vi "Get Table Data.vi"(7 "Count? (F)":bool, 8 "error in (no error)":errorcluster, 9 "Column Conditions[] (Optional)":T1[](array[typedef]), 10 "Header Order[] (Optional)":string[](array[string]), 11 "SLL Table in":refnum<class "SLL Table.lvclass">) -> (0 "error out":errorcluster, 1 "2D Data Out[][]":string[][](array[string]), 2 "Headers Out[]":string[](array[string]), 3 "SLL Table out":refnum<class "SLL Table.lvclass">)   [LabVIEW 2014, in "SLL Table.lvclass"]
doc: "Get the data that you need & in the column order you want. \n\nYou can specify the column header and the value as conditions."
uses:
  SLL Table.lvclass
  _Typedefs/ColumnConditionCluster.ctl
  <userlib>/_OpenG.lib/array/array.llb/Remove Duplicates from 1D Array (String)__ogtk.vi
  SLL String/SLL String.lvlib
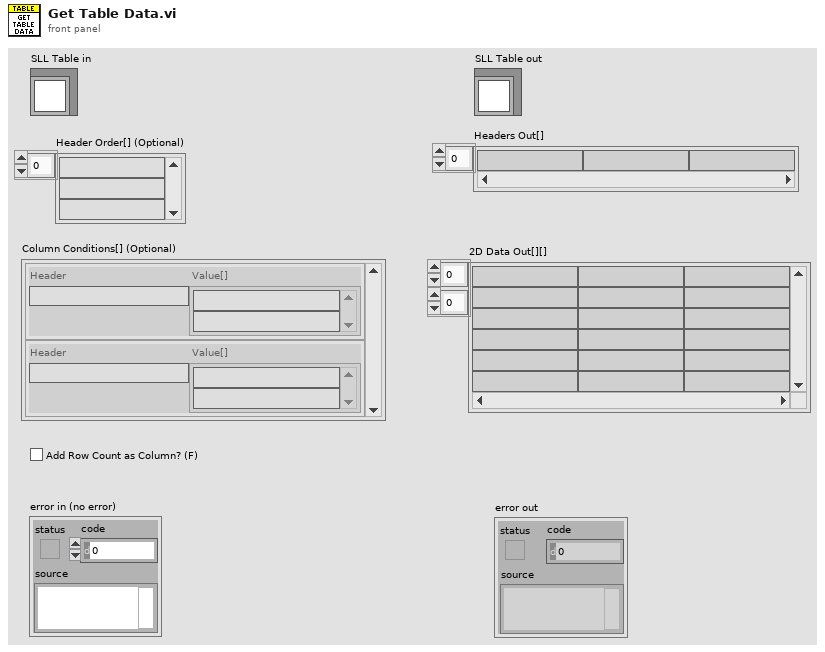
[diagram p1: front panel]
types:
  T1 = typedef "ColumnConditionCluster.ctl" = cluster{"Header":string, "Value[]":string[]}
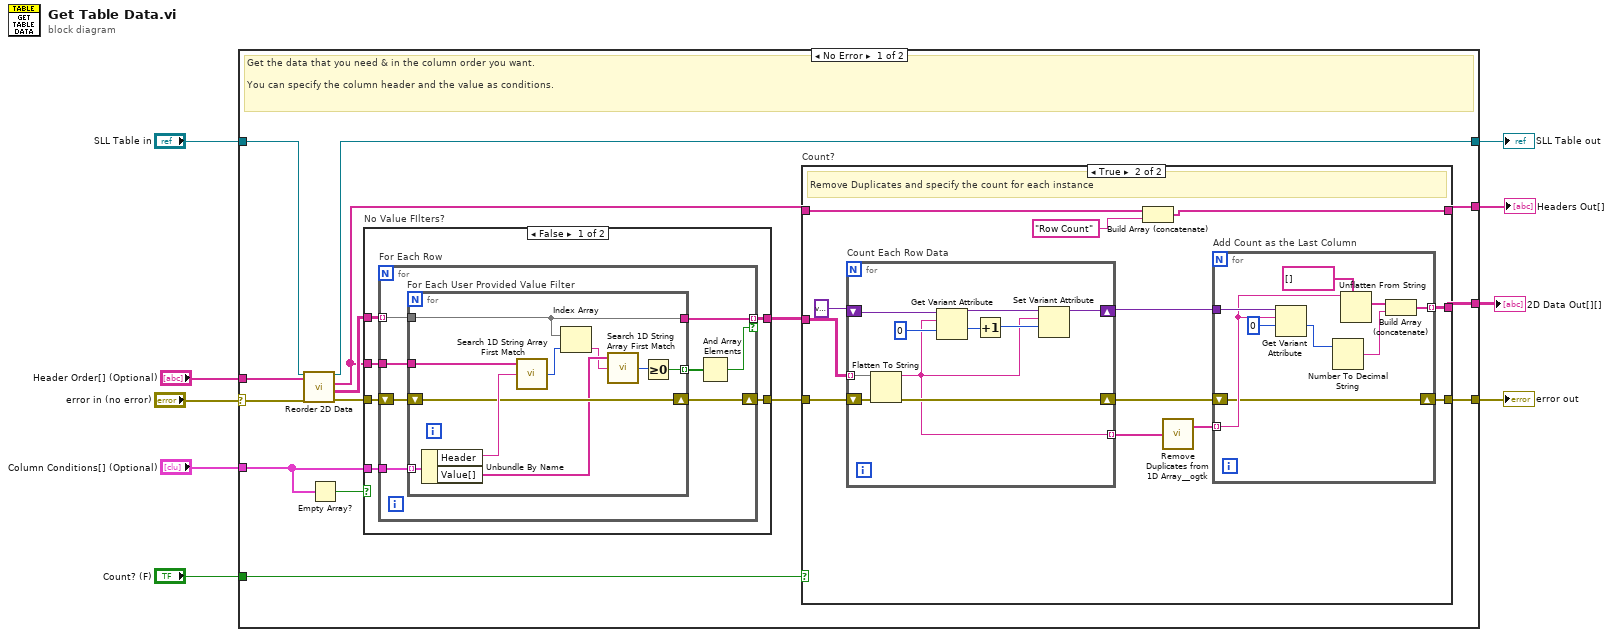
[diagram p0: block diagram]
diagram:
  n1 = case shown="No Error" "error in (no error)" {
    selector: "error in (no error)" -> [w24 w86]
    tunnel: [w13 w86] -> w8
    tunnel: [w22 w85] -> w6
    tunnel: "SLL Table in" -> [w23 w85]
    tunnel: "Header Order[] (Optional)" -> [w21 _]
    tunnel: [w20 _] -> w4
    tunnel: [w19 _] -> w3
    tunnel: "Column Conditions[] (Optional)" -> [w16 _]
    tunnel: "Count? (F)" -> [w12 _]
    frame No Error {
      # "Get the data that you need & in the column order you want. \n\nYou can specify the column header and the value as conditions."
      n2 = call "Reorder 2D Data.vi"("error in (no error)"=w24, "Header Order[]"=w21, "SLL Table in"=w23) -> ("error out"=w11:errorcluster, "2D Data Out[][]"=w18:string[][], "Headers Out[]"=w14:string[], "SLL Table out"=w22:refnum<class "SLL Table.lvclass">)  [unwired: 5 in]
      n3 = Empty Array?(array=w16) -> (empty?=w17:bool)
      n4 = case "No Value FIlters?" shown="False" w17 {
        tunnel: w18 -> [w64 w84]
        tunnel: w14 -> [w63 _]
        tunnel: w16 -> [w62 _]
        tunnel: [w61 w84] -> w15
        tunnel: w11 -> [w60 w83]
        tunnel: [w59 w83] -> w10
        frame False {
          n5 = for "For Each Row" {
            tunnel: w64 -> [w71] mode=indexing
            tunnel: w63 -> [w70]
            tunnel: w62 -> [w72]
            tunnel: [w69] -> w61 mode=indexing if=w67
            shift-right: [w65] -> w59
            shift-left: w60 -> [w66]
            n6 = for "For Each User Provided Value Filter" {
              tunnel: w72 -> [w82] mode=indexing
              tunnel: w71 -> [w78]
              tunnel: w70 -> [w81]
              tunnel: [w73] -> w68 mode=indexing
              tunnel: [w78] -> w69
              shift-right: [w77] -> w65
              shift-left: w66 -> [w77]
              n7 = Unbundle By Name(w82) -> ("Header"=w80:string, "Value[]"=w76:string[])
              n8 = call "Search 1D String Array First Match.vi"("Element"=w80, "1D String Array"=w81) -> ("Index"=w79:i32)  [unwired: 1 in]
              n9 = Index Array(array=w78, index=w79) -> (element=w75:string)
              n10 = call "Search 1D String Array First Match.vi"("Element"=w75, "1D String Array"=w76) -> ("Index"=w74:i32)  [unwired: 1 in]
              n11 = Greater Or Equal To 0?(x=w74) -> (x >= 0?=w73:bool)
            }
            n12 = And Array Elements(Boolean array=w68) -> (logical AND=w67:bool)
          }
        }
        frame True {
          # "No Value Filters"
        }
      }
      n13 = case "Count?" shown="True" w12 {
        tunnel: [w27 w36] -> w20
        tunnel: [w26 w35] -> w19
        tunnel: w15 -> [w26 w33]
        tunnel: w14 -> [w27 w32]
        tunnel: [w25 w29] -> w13
        tunnel: w10 -> [w25 w28]
        frame False {
        }
        frame True {
          # "Remove Duplicates and specify the count for each instance"
          n14 = for "Count Each Row Data" {
            shift-right: [w55] -> w38
            shift-left: variant -> [w58]
            tunnel: w33 -> [w54] mode=indexing
            shift-right: [w50] -> w30
            shift-left: w28 -> [w51]
            tunnel: [w49] -> w34 mode=indexing
            n15 = Flatten To String(anything=w54, error in (no error)=w51) -> (data string=w49:string, error out=w50:errorcluster)  [unwired: 2 in, 1 out]
            n16 = Get Variant Attribute(Variant=w58, name=w49, default value (empty Variant)=0) -> (duplicate Variant=w56:variant, value=w53:i32)  [unwired: 1 in, 2 out]
            n17 = Increment(x=w53) -> (x+1=w52:i32)
            n18 = Set Variant Attribute(Variant=w56, name=w49, value=w52) -> (Variant out=w55:variant)  [unwired: 1 in, 2 out]
          }
          n19 = Build Array (concatenate)(w32, "Row Count") -> (w36:string[])
          n20 = call-poly <userlib>:"Remove Duplicates from 1D Array__ogtk.vi"("Input Array"=w34) -> ("Output Array"=w31:string[])  [unwired: 1 out]
          n21 = for "Add Count as the Last Column" {
            tunnel: w38 -> [w48]
            tunnel: w31 -> [w44] mode=indexing
            tunnel: [w41] -> w35 mode=indexing
            shift-right: [w40] -> w29
            shift-left: w30 -> [w40]
            n22 = Get Variant Attribute(Variant=w48, name=w44, default value (empty Variant)=0) -> (value=w46:i32)  [unwired: 1 in, 3 out]
            n23 = Number To Decimal String(number=w46) -> (decimal integer string=w42:string)  [unwired: 1 in]
            n24 = Unflatten From String(type=string[] [] ("2D Data Out[][]"), binary string=w44) -> (value=w43:string[])  [unwired: 3 in, 2 out]
            n25 = Build Array (concatenate)(w43, w42) -> (w41:string[])
          }
        }
      }
    }
    frame Error {
    }
  }
  "error out" <- w8
  "SLL Table out" <- w6
  "2D Data Out[][]" <- w3
  "Headers Out[]" <- w4
